vi "Retrieve Table (string).vi"(8 "error in (no error)":errorcluster, 11 "Document in":refnum<class "Document.lvclass">) -> (0 "error out":errorcluster, 2 "Table":string[][](array[string]), 3 "Document out":refnum<class "Document.lvclass">)   [LabVIEW 2017, in "LabVIEW NPOI.lvlib" / "Document.lvclass"]
doc: "Returns the <b>Table</b> as 2D array of strings from the <b>Document</b> as a table."
uses:
  Document.lvclass
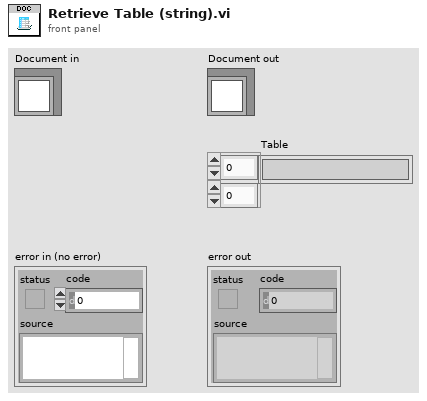
[diagram p1: front panel]
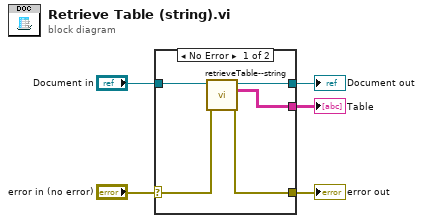
[diagram p0: block diagram]
diagram:
  n1 = case shown="No Error" "error in (no error)" {
    selector: "error in (no error)" -> [w7 w12]
    tunnel: [w6 w12] -> w4
    tunnel: [w9 w11] -> w2
    tunnel: "Document in" -> [w10 w11]
    tunnel: [w8 _] -> w1
    frame No Error {
      n2 = call-dynamic "retrieveTable--string.vi"("error in (no error)"=w7, "Document in"=w10) -> ("error out"=w6:errorcluster, "Table"=w8:string[][], "Document out"=w9:refnum<class "Document.lvclass">)  [unwired: 7 in]
    }
    frame Error {
    }
  }
  "error out" <- w4
  "Document out" <- w2
  "Table" <- w1
